vi "CVT Globals.vi"() -> ()   [LabVIEW 2020, in "Current Value Table(Rebuild).lvlib"]
uses:
  Current Value Table(Rebuild).lvlib
panel:
  out "Reset count":u32
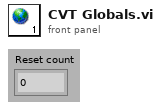
[diagram p1: front panel]
diagram:
